vi "MouseFocus.vi"(2 "Image Settings":T1, 3 "mouse focus":cluster{"device ID":refnum<k1>, "Scrolling":i32}, 4 "Position increment":refnum<vi>) -> (0 "mouse focus":cluster{"device ID":refnum<k1>, "Scrolling":i32}, 1 "Image Settings":T1)   [LabVIEW 2009]
uses:
  <vilib>/Utility/inputDevices.llb/mouseAcquire.vi
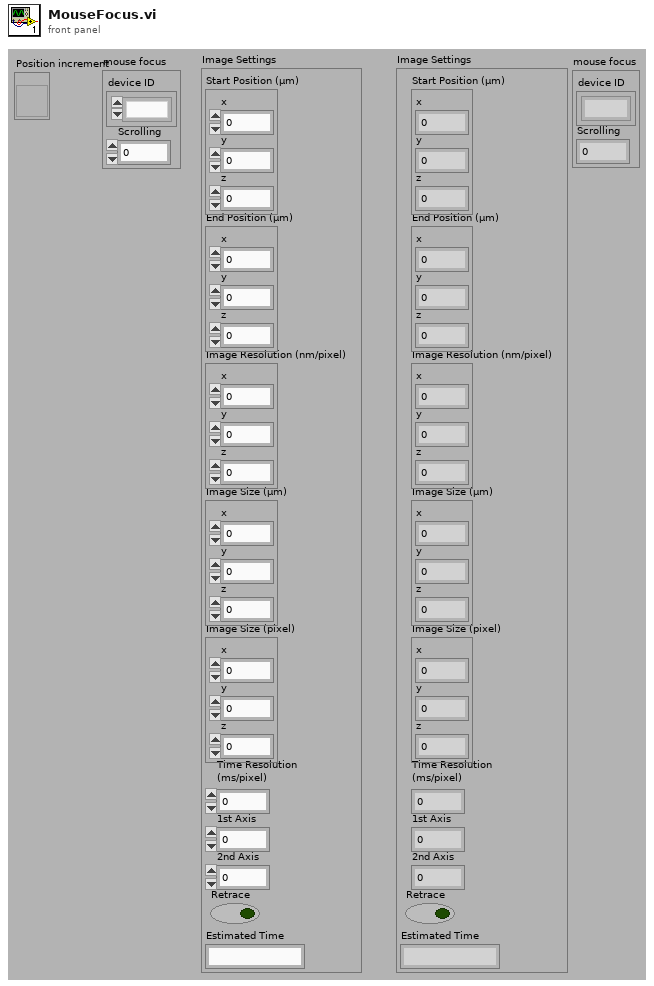
[diagram p1: front panel]
types:
  T1 = cluster{"Start Position (µm)":cluster{"x":dbl, "y":dbl, "z":dbl}, "End Position (µm)":cluster{"x":dbl, "y":dbl, "z":dbl}, "Image Resolution (nm/pixel)":cluster{"x":dbl, "y":dbl, "z":dbl}, "Image Size (µm)":cluster{"x":dbl, "y":dbl, "z":dbl}, "Image Size (pixel)":cluster{"x":u32, "y":u32, "z":u32}, "Time Resolution\n(ms/pixel)":dbl, "1st Axis":u16, "2nd Axis":u16, "Retrace":bool, "Estimated Time":string}
  T2 = cluster{"Horizontal":i32, "Vertical":i32, "Scrolling":i32}
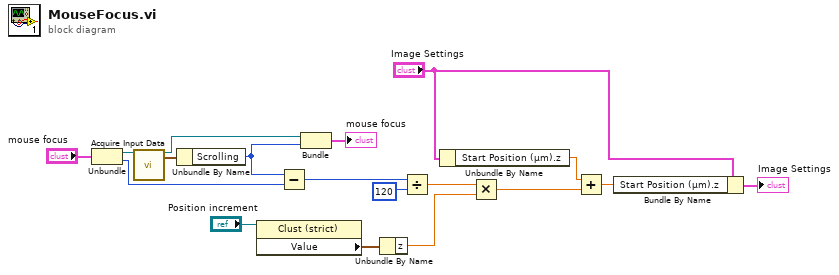
[diagram p0: block diagram]
diagram:
  n1 = Unbundle("mouse focus") -> ("device ID"=w13:refnum<k1>, "Scrolling"=w14:i32)
  n2 = call-poly <vilib>:"Acquire Input Data.vi"("device ID"=w13) -> ("device ID"=w15:refnum<k1>, "axis info"=w2:T2)  [unwired: 15 in, 2 out]
  n3 = Unbundle By Name(w2) -> ("Scrolling"=w18:i32)
  n4 = property on="Property Node" class="Clust (strict)"(reference="Position increment") -> ("Value"=w4:cluster{"x":dbl, "y":dbl, "z":dbl})  [unwired: 1 in, 2 out]
  n5 = Subtract(x=w18, y=w14) -> (x-y=w16:i32)
  n6 = Bundle("device ID"=w15, "Scrolling"=w18) -> (→"mouse focus":cluster{"device ID":refnum<k1>, "Scrolling":i32})  [unwired: 1 in]
  n7 = Unbundle By Name(w4) -> ("z"=w6:dbl)
  n8 = Divide(x=w16, y=120) -> (x/y=w5:dbl)
  n9 = Unbundle By Name("Image Settings") -> ("Start Position (µm).z"=w7:dbl)
  n10 = Multiply(x=w5, y=w6) -> (x*y=w8:dbl)
  n11 = Add(x=w7, y=w8) -> (x+y=w10:dbl)
  n12 = Bundle By Name(cluster="Image Settings", "Start Position (µm).z"=w10) -> (→"Image Settings":T1)
